vi "Calculate T from Rt using SHH.vi"(10 "R":dbl[](array[numeric]), 11 "Coefficients":dbl[](array[numeric])) -> (3 "Array":dbl[](array[numeric]))   [LabVIEW 2015, in "Temperature.lvlib"]
uses:
  Temperature.lvlib
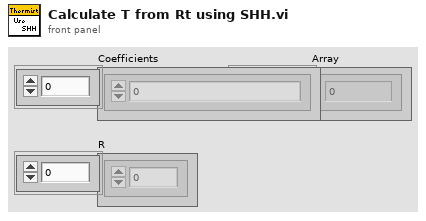
[diagram p1: front panel]
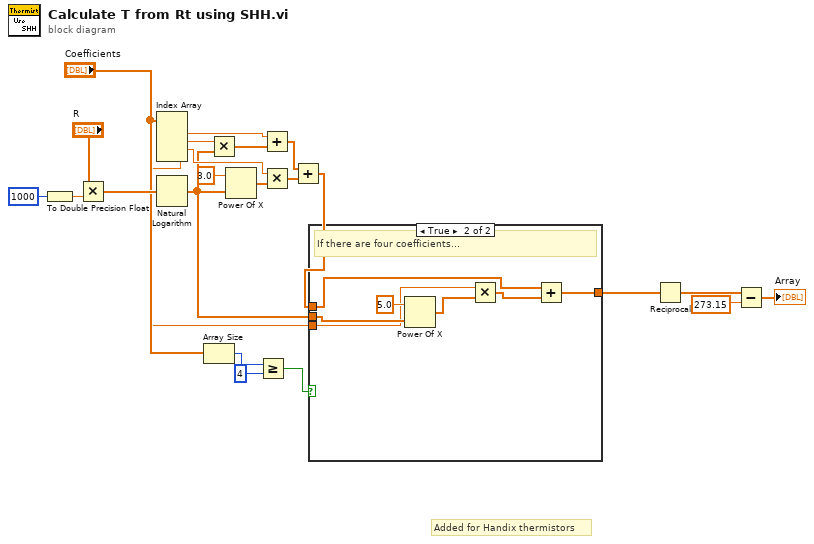
[diagram p0: block diagram]
diagram:
  # "Added for Handix thermistors"
  n1 = To Double Precision Float(number=1000) -> (double precision float=w23:dbl)
  n2 = Multiply(x="R", y=w23) -> (x*y=w21:dbl[])
  n3 = Index Array(array="Coefficients") -> (element #1=w9:dbl, element #2=w11:dbl, element #3=w13:dbl, element #4=w5:dbl)  [unwired: 4 in]
  n4 = Natural Logarithm(1:w21) -> (0:w3:dbl[])
  n5 = Array Size(array="Coefficients") -> (size(s)=w7:i32)
  n6 = Multiply(x=w11, y=w3) -> (x*y=w12:dbl[])
  n7 = Power Of X(1:w3, 2:3.0 ("y")) -> (0:w14:dbl[])
  n8 = Greater Or Equal?(x=w7, y=4) -> (x >= y?=w1:bool)
  n9 = Add(x=w9, y=w12) -> (x+y=w16:dbl[])
  n10 = Multiply(x=w13, y=w14) -> (x*y=w15:dbl[])
  n11 = Add(x=w16, y=w15) -> (x+y=w4:dbl[])
  n12 = case shown="True" w1 {
    tunnel: w5 -> [_ w28]
    tunnel: w4 -> [w24 w26]
    tunnel: w3 -> [_ w30]
    tunnel: [w24 w25] -> w2
    frame False {
    }
    frame True {
      # "If there are four coefficients..."
      n13 = Power Of X(1:w30, 2:5.0 ("y")) -> (0:w29:dbl[])
      n14 = Multiply(x=w28, y=w29) -> (x*y=w27:dbl[])
      n15 = Add(x=w26, y=w27) -> (x+y=w25:dbl[])
    }
  }
  n16 = Reciprocal(x=w2) -> (1/x=w17:dbl[])
  n17 = Subtract(x=w17, y=273.15) -> (x-y=→"Array":dbl[])
